vi "Distance calculation.vi"(8 "look up table":string[][](array[string])=[["", "1 0", "0 1", "1 -1", "-1 1", "1 -4", "-4 1", "2 0", "0 2", "2 -1", "-1 2", "2 -2", "-2 2", "3 0", "0 3", "3 -2", "-2 3", "3 -3", "-3 3", "4 0", "0 4", "4 -3", "-3 4", "4 -4", "-4 4", "-1 0", "0 -1", "-2 0", "0 -2", "-3 0", "0 -3", "-4 0", "0 -4", "-1 -2", "-2 -1", "-2 -3", "-3 -2", "-3 -4", "-4 -3", "-4 -1", "-1 -4"], ["-4", "2", "2", "2", "2", "1", "0", "4", "4", "4", "4", "4", "4", "4", "4", "4", "4", "4", "4", "2", "2", "2", "2", "1", "0", "3", "2", "5", "5", "3", "2", "0", "1", "4", "4", "4", "4", "1", "0", "0", "1"], ["-3", "4", "4", "4", "4", "4", "4", "4", "4", "4", "4", "4", "4", "2", "2", "2", "2", "1", "0", "2", "2", "1", "0", "2", "2", "5", "5", "3", "2", "0", "1", "3", "2", "4", "4", "1", "0", "0", "1", "4", "4"], ["-2", "4", "4", "4", "4", "4", "4", "2", "2", "2", "2", "1", "0", "2", "2", "1", "0", "2", "2", "4", "4", "4", "4", "4", "4", "3", "2", "0", "1", "3", "2", "5", "5", "1", "0", "0", "1", "4", "4", "4", "4"], ["-1", "2", "2", "1", "0", "2", "2", "2", "2", "1", "0", "2", "2", "4", "4", "4", "4", "4", "4", "4", "4", "4", "4", "4", "4", "0", "1", "3", "2", "5", "5", "3", "2", "0", "1", "4", "4", "4", "4", "1", "0"], ["0", "1", "0", "2", "2", "2", "2", "1", "0", "2", "2", "2", "2", "1", "0", "2", "2", "2", "2", "1", "0", "2", "2", "2", "2", "1", "0", "1", "0", "1", "0", "1", "0", "2", "2", "2", "2", "2", "2", "2", "2"], ["1", "0", "1", "0", "1", "0", "1", "3", "3", "3", "3", "3", "3", "5", "5", "5", "5", "5", "5", "3", "3", "3", "3", "3", "3", "2", "3", "4", "4", "4", "4", "2", "3", "3", "3", "5", "5", "3", "3", "2", "2"], ["2", "3", "3", "3", "3", "3", "3", "0", "1", "0", "1", "0", "1", "3", "3", "3", "3", "3", "3", "5", "5", "5", "5", "5", "5", "2", "3", "2", "3", "4", "4", "4", "4", "2", "2", "3", "3", "5", "5", "3", "3"], ["3", "5", "5", "5", "5", "5", "5", "3", "3", "3", "3", "3", "3", "0", "1", "0", "1", "0", "1", "3", "3", "3", "3", "3", "3", "4", "4", "2", "3", "2", "3", "4", "4", "3", "3", "2", "2", "3", "3", "5", "5"], ["4", "3", "3", "3", "3", "3", "3", "5", "5", "5", "5", "5", "5", "3", "3", "3", "3", "3", "3", "0", "1", "0", "1", "0", "1", "4", "4", "4", "4", "2", "3", "2", "3", "5", "5", "3", "3", "4", "4", "3", "3"]], 10 "cluster centers":string[](array[string])=["1 0 1", "2 0 2", "3 0 3", "4 0 4"], 11 "Patterns in":string[](array[string])=["0 4 0", "4 0 4", "0 4 0", "4 0 4", "0 4 0", "4 0 4", "0 4 0", "4 0 -2", "0 -2 3", "-2 3 0", "3 0 3", "0 3 0", "3 0 4", "0 4 0", "-2 0 1", "0 1 0", "1 0 -4", "0 -4 4", "-2 2 0", "2 0 -1", "0 -1 -4", "-1 -4 1", "-4 1 0", "1 0 3", "0 3 0", "-1 0 -1", "0 -1 2", "0 -1 1", "-1 1 0", "1 0 4", "0 4 0", "4 0 3", "0 3 -2", "3 -2 0", "-2 0 -2", "0 -2 3", "-2 3 -2", "3 -2 0", "-2 0 4", "0 4 0", "4 0 -2", "0 -2 2", "2 -1 0", "-1 0 4", "0 4 0", "4 0 2", "0 2 0", "2 0 -2", "0 -2 0", "1 -1 0", "-1 0 3", "0 3 0", "3 0 -4", "0 -4 4", "-4 4 -4", "4 -4 0", "2 -1 0", "-1 0 3", "0 3 -2", "3 -2 0", "-2 0 -3", "0 -3 0", "-3 0 3", "0 3 0", "3 0 -3", "0 -3 0", "0 4 0", "4 0 4", "0 4 -4", "4 -4 1", "-4 1 -1", "1 -1 0", "-1 0 -3", "0 -3 0", "-3 0 1", "0 1 -4", "1 -4 1", "-4 1 0", "1 0 4", "0 4 0", "4 0 -4", "0 -4 0", "-4 0 -4", "0 -4 4", "-4 4 -4", "4 -4 1", "0 -4 1", "-4 1 0", "1 0 -4", "0 -4 4", "0 4 0", "4 0 -2", "0 -2 2", "-2 2 -2", "2 -2 2", "-2 2 -2", "2 -2 2", "-2 2 -1", "2 -1 0", "-1 0 4", "0 4 0", "4 0 2", "0 2 0", "2 0 4", "0 4 0", "4 0 2", "0 2 -2", "2 -2 0", "-2 0 4", "1 0 -1", "0 -1 0", "-1 0 -1", "0 -1 0", "-1 0 1", "0 1 -1", "-2 2 -2", "2 -2 3", "1 0 -1", "0 -1 0", "-1 0 -1", "0 -1 2", "-1 2 0", "2 0 2", "0 2 -2", "2 -2 0", "-2 0 -4", "0 -4 0", "-2 2 0", "2 0 3", "0 3 -2", "3 -2 2", "1 -1 0", "-1 0 3", "0 4 0", "-2 0 1", "0 1 -4", "1 -4 0", "-4 0 -3", "0 -3 0", "1 0 -1", "0 -1 2", "-1 2 -1", "2 -1 1", "-1 1 -4", "-2 0 -1", "0 -1 1", "0 3 0", "3 0 3", "0 3 0", "3 0 3", "0 3 -2", "-4 0 -4", "0 -4 4", "0 4 0", "4 0 -4", "0 -4 0", "-4 0 -4", "-2 2 0", "2 0 4", "0 4 -4", "4 -4 0", "-4 0 2", "0 2 -2"]) -> (3 "Pattern (0) Distance data (1 to X) cluster (X+1) output":string[][](array[string]))   [LabVIEW 2013]
uses:
  cluster.ctl
panel:
  in  "15":string[](array[string])=["0 4 0 4 0 4 0 4 0 -2 3 0 3 0 4", "4 0 4 0 4 0 4 0 -2 3 0 3 0 4 0", "0 -1 1 0 4 0 3 -2 0 -2 3 -2 0 4 0", "-1 1 0 4 0 3 -2 0 -2 3 -2 0 4 0 -2", "1 0 4 0 3 -2 0 -2 3 -2 0 4 0 -2 2", "0 4 0 4 -4 1 -1 0 -3 0 1 -4 1 0 4", "4 0 4 -4 1 -1 0 -3 0 1 -4 1 0 4 0", "0 4 -4 1 -1 0 -3 0 1 -4 1 0 4 0 -4", "4 -4 1 -1 0 -3 0 1 -4 1 0 4 0 -4 0", "-4 1 -1 0 -3 0 1 -4 1 0 4 0 -4 0 -4", "1 -1 0 -3 0 1 -4 1 0 4 0 -4 0 -4 4", "-1 0 -3 0 1 -4 1 0 4 0 -4 0 -4 4 -4", "0 -3 0 1 -4 1 0 4 0 -4 0 -4 4 -4 1"]
  in  "14":string[](array[string])=["0 4 0 4 0 4 0 4 0 -2 3 0 3 0", "4 0 4 0 4 0 4 0 -2 3 0 3 0 4", "0 4 0 4 0 4 0 -2 3 0 3 0 4 0", "0 -1 1 0 4 0 3 -2 0 -2 3 -2 0 4", "-1 1 0 4 0 3 -2 0 -2 3 -2 0 4 0", "1 0 4 0 3 -2 0 -2 3 -2 0 4 0 -2", "0 4 0 3 -2 0 -2 3 -2 0 4 0 -2 2", "0 4 0 4 -4 1 -1 0 -3 0 1 -4 1 0", "4 0 4 -4 1 -1 0 -3 0 1 -4 1 0 4", "0 4 -4 1 -1 0 -3 0 1 -4 1 0 4 0", "4 -4 1 -1 0 -3 0 1 -4 1 0 4 0 -4", "-4 1 -1 0 -3 0 1 -4 1 0 4 0 -4 0", "1 -1 0 -3 0 1 -4 1 0 4 0 -4 0 -4", "-1 0 -3 0 1 -4 1 0 4 0 -4 0 -4 4", "0 -3 0 1 -4 1 0 4 0 -4 0 -4 4 -4", "-3 0 1 -4 1 0 4 0 -4 0 -4 4 -4 1", "-2 2 -1 0 4 0 2 0 4 0 2 -2 0 4"]
  in  "11":string[](array[string])=["0 4 0 4 0 4 0 4 0 -2 3", "4 0 4 0 4 0 4 0 -2 3 0", "0 4 0 4 0 4 0 -2 3 0 3", "4 0 4 0 4 0 -2 3 0 3 0", "0 4 0 4 0 -2 3 0 3 0 4", "4 0 4 0 -2 3 0 3 0 4 0", "0 -1 1 0 4 0 3 -2 0 -2 3", "-1 1 0 4 0 3 -2 0 -2 3 -2", "1 0 4 0 3 -2 0 -2 3 -2 0", "0 4 0 3 -2 0 -2 3 -2 0 4", "4 0 3 -2 0 -2 3 -2 0 4 0", "0 3 -2 0 -2 3 -2 0 4 0 -2", "3 -2 0 -2 3 -2 0 4 0 -2 2", "2 -1 0 3 -2 0 -3 0 3 0 -3", "-1 0 3 -2 0 -3 0 3 0 -3 0", "0 4 0 4 -4 1 -1 0 -3 0 1", "4 0 4 -4 1 -1 0 -3 0 1 -4", "0 4 -4 1 -1 0 -3 0 1 -4 1", "4 -4 1 -1 0 -3 0 1 -4 1 0", "-4 1 -1 0 -3 0 1 -4 1 0 4", "1 -1 0 -3 0 1 -4 1 0 4 0", "-1 0 -3 0 1 -4 1 0 4 0 -4", "0 -3 0 1 -4 1 0 4 0 -4 0", "-3 0 1 -4 1 0 4 0 -4 0 -4", "0 1 -4 1 0 4 0 -4 0 -4 4", "1 -4 1 0 4 0 -4 0 -4 4 -4", "-4 1 0 4 0 -4 0 -4 4 -4 1", "-2 2 -1 0 4 0 2 0 4 0 2", "2 -1 0 4 0 2 0 4 0 2 -2", "-1 0 4 0 2 0 4 0 2 -2 0", "0 4 0 2 0 4 0 2 -2 0 4", "1 0 -1 0 -1 2 0 2 -2 0 -4", "0 -1 0 -1 2 0 2 -2 0 -4 0"]
  in  "10":string[](array[string])=["0 4 0 4 0 4 0 4 0 -2", "4 0 4 0 4 0 4 0 -2 3", "0 4 0 4 0 4 0 -2 3 0", "4 0 4 0 4 0 -2 3 0 3", "0 4 0 4 0 -2 3 0 3 0", "4 0 4 0 -2 3 0 3 0 4", "0 4 0 -2 3 0 3 0 4 0", "0 -1 1 0 4 0 3 -2 0 -2", "-1 1 0 4 0 3 -2 0 -2 3", "1 0 4 0 3 -2 0 -2 3 -2", "0 4 0 3 -2 0 -2 3 -2 0", "4 0 3 -2 0 -2 3 -2 0 4", "0 3 -2 0 -2 3 -2 0 4 0", "3 -2 0 -2 3 -2 0 4 0 -2", "-2 0 -2 3 -2 0 4 0 -2 2", "2 -1 0 3 -2 0 -3 0 3 0", "-1 0 3 -2 0 -3 0 3 0 -3", "0 3 -2 0 -3 0 3 0 -3 0", "0 4 0 4 -4 1 -1 0 -3 0", "4 0 4 -4 1 -1 0 -3 0 1", "0 4 -4 1 -1 0 -3 0 1 -4", "4 -4 1 -1 0 -3 0 1 -4 1", "-4 1 -1 0 -3 0 1 -4 1 0", "1 -1 0 -3 0 1 -4 1 0 4", "-1 0 -3 0 1 -4 1 0 4 0", "0 -3 0 1 -4 1 0 4 0 -4", "-3 0 1 -4 1 0 4 0 -4 0", "0 1 -4 1 0 4 0 -4 0 -4", "1 -4 1 0 4 0 -4 0 -4 4", "-4 1 0 4 0 -4 0 -4 4 -4", "1 0 4 0 -4 0 -4 4 -4 1", "-2 2 -1 0 4 0 2 0 4 0", "2 -1 0 4 0 2 0 4 0 2", "-1 0 4 0 2 0 4 0 2 -2", "0 4 0 2 0 4 0 2 -2 0", "4 0 2 0 4 0 2 -2 0 4", "1 0 -1 0 -1 2 0 2 -2 0", "0 -1 0 -1 2 0 2 -2 0 -4", "-1 0 -1 2 0 2 -2 0 -4 0"]
  in  "9":string[](array[string])=["0 4 0 4 0 4 0 4 0", "4 0 4 0 4 0 4 0 -2", "0 4 0 4 0 4 0 -2 3", "4 0 4 0 4 0 -2 3 0", "0 4 0 4 0 -2 3 0 3", "4 0 4 0 -2 3 0 3 0", "0 4 0 -2 3 0 3 0 4", "4 0 -2 3 0 3 0 4 0", "-2 2 0 -1 -4 1 0 3 0", "0 -1 1 0 4 0 3 -2 0", "-1 1 0 4 0 3 -2 0 -2", "1 0 4 0 3 -2 0 -2 3", "0 4 0 3 -2 0 -2 3 -2", "4 0 3 -2 0 -2 3 -2 0", "0 3 -2 0 -2 3 -2 0 4", "3 -2 0 -2 3 -2 0 4 0", "-2 0 -2 3 -2 0 4 0 -2", "0 -2 3 -2 0 4 0 -2 2", "1 -1 0 3 0 -4 4 -4 0", "2 -1 0 3 -2 0 -3 0 3", "-1 0 3 -2 0 -3 0 3 0", "0 3 -2 0 -3 0 3 0 -3", "3 -2 0 -3 0 3 0 -3 0", "0 4 0 4 -4 1 -1 0 -3", "4 0 4 -4 1 -1 0 -3 0", "0 4 -4 1 -1 0 -3 0 1", "4 -4 1 -1 0 -3 0 1 -4", "-4 1 -1 0 -3 0 1 -4 1", "1 -1 0 -3 0 1 -4 1 0", "-1 0 -3 0 1 -4 1 0 4", "0 -3 0 1 -4 1 0 4 0", "-3 0 1 -4 1 0 4 0 -4", "0 1 -4 1 0 4 0 -4 0", "1 -4 1 0 4 0 -4 0 -4", "-4 1 0 4 0 -4 0 -4 4", "1 0 4 0 -4 0 -4 4 -4", "0 4 0 -4 0 -4 4 -4 1", "0 4 0 -2 2 -2 2 -2 2", "-2 2 -1 0 4 0 2 0 4", "2 -1 0 4 0 2 0 4 0", "-1 0 4 0 2 0 4 0 2", "0 4 0 2 0 4 0 2 -2", "4 0 2 0 4 0 2 -2 0", "0 2 0 4 0 2 -2 0 4", "1 0 -1 0 -1 2 0 2 -2", "0 -1 0 -1 2 0 2 -2 0", "-1 0 -1 2 0 2 -2 0 -4", "0 -1 2 0 2 -2 0 -4 0"]
  in  "8":string[](array[string])=["0 4 0 4 0 4 0 4", "4 0 4 0 4 0 4 0", "0 4 0 4 0 4 0 -2", "4 0 4 0 4 0 -2 3", "0 4 0 4 0 -2 3 0", "4 0 4 0 -2 3 0 3", "0 4 0 -2 3 0 3 0", "4 0 -2 3 0 3 0 4", "0 -2 3 0 3 0 4 0", "-2 2 0 -1 -4 1 0 3", "2 0 -1 -4 1 0 3 0", "0 -1 1 0 4 0 3 -2", "-1 1 0 4 0 3 -2 0", "1 0 4 0 3 -2 0 -2", "0 4 0 3 -2 0 -2 3", "4 0 3 -2 0 -2 3 -2", "0 3 -2 0 -2 3 -2 0", "3 -2 0 -2 3 -2 0 4", "-2 0 -2 3 -2 0 4 0", "0 -2 3 -2 0 4 0 -2", "-2 3 -2 0 4 0 -2 2", "1 -1 0 3 0 -4 4 -4", "-1 0 3 0 -4 4 -4 0", "2 -1 0 3 -2 0 -3 0", "-1 0 3 -2 0 -3 0 3", "0 3 -2 0 -3 0 3 0", "3 -2 0 -3 0 3 0 -3", "-2 0 -3 0 3 0 -3 0", "0 4 0 4 -4 1 -1 0", "4 0 4 -4 1 -1 0 -3", "0 4 -4 1 -1 0 -3 0", "4 -4 1 -1 0 -3 0 1", "-4 1 -1 0 -3 0 1 -4", "1 -1 0 -3 0 1 -4 1", "-1 0 -3 0 1 -4 1 0", "0 -3 0 1 -4 1 0 4", "-3 0 1 -4 1 0 4 0", "0 1 -4 1 0 4 0 -4", "1 -4 1 0 4 0 -4 0", "-4 1 0 4 0 -4 0 -4", "1 0 4 0 -4 0 -4 4", "0 4 0 -4 0 -4 4 -4", "4 0 -4 0 -4 4 -4 1", "0 4 0 -2 2 -2 2 -2", "4 0 -2 2 -2 2 -2 2", "-2 2 -1 0 4 0 2 0", "2 -1 0 4 0 2 0 4", "-1 0 4 0 2 0 4 0", "0 4 0 2 0 4 0 2", "4 0 2 0 4 0 2 -2", "0 2 0 4 0 2 -2 0", "2 0 4 0 2 -2 0 4", "1 0 -1 0 -1 0 1 -1", "1 0 -1 0 -1 2 0 2", "0 -1 0 -1 2 0 2 -2", "-1 0 -1 2 0 2 -2 0", "0 -1 2 0 2 -2 0 -4", "-1 2 0 2 -2 0 -4 0", "-2 2 0 4 -4 0 2 -2"]
  in  "7":string[](array[string])=["0 4 0 4 0 4 0", "4 0 4 0 4 0 4", "0 4 0 4 0 4 0", "4 0 4 0 4 0 -2", "0 4 0 4 0 -2 3", "4 0 4 0 -2 3 0", "0 4 0 -2 3 0 3", "4 0 -2 3 0 3 0", "0 -2 3 0 3 0 4", "-2 3 0 3 0 4 0", "-2 2 0 -1 -4 1 0", "2 0 -1 -4 1 0 3", "0 -1 -4 1 0 3 0", "0 -1 1 0 4 0 3", "-1 1 0 4 0 3 -2", "1 0 4 0 3 -2 0", "0 4 0 3 -2 0 -2", "4 0 3 -2 0 -2 3", "0 3 -2 0 -2 3 -2", "3 -2 0 -2 3 -2 0", "-2 0 -2 3 -2 0 4", "0 -2 3 -2 0 4 0", "-2 3 -2 0 4 0 -2", "3 -2 0 4 0 -2 2", "0 4 0 2 0 -2 0", "1 -1 0 3 0 -4 4", "-1 0 3 0 -4 4 -4", "0 3 0 -4 4 -4 0", "2 -1 0 3 -2 0 -3", "-1 0 3 -2 0 -3 0", "0 3 -2 0 -3 0 3", "3 -2 0 -3 0 3 0", "-2 0 -3 0 3 0 -3", "0 -3 0 3 0 -3 0", "0 4 0 4 -4 1 -1", "4 0 4 -4 1 -1 0", "0 4 -4 1 -1 0 -3", "4 -4 1 -1 0 -3 0", "-4 1 -1 0 -3 0 1", "1 -1 0 -3 0 1 -4", "-1 0 -3 0 1 -4 1", "0 -3 0 1 -4 1 0", "-3 0 1 -4 1 0 4", "0 1 -4 1 0 4 0", "1 -4 1 0 4 0 -4", "-4 1 0 4 0 -4 0", "1 0 4 0 -4 0 -4", "0 4 0 -4 0 -4 4", "4 0 -4 0 -4 4 -4", "0 -4 0 -4 4 -4 1", "0 4 0 -2 2 -2 2", "4 0 -2 2 -2 2 -2", "0 -2 2 -2 2 -2 2", "-2 2 -1 0 4 0 2", "2 -1 0 4 0 2 0", "-1 0 4 0 2 0 4", "0 4 0 2 0 4 0", "4 0 2 0 4 0 2", "0 2 0 4 0 2 -2", "2 0 4 0 2 -2 0", "0 4 0 2 -2 0 4", "1 0 -1 0 -1 0 1", "0 -1 0 -1 0 1 -1", "1 0 -1 0 -1 2 0", "0 -1 0 -1 2 0 2", "-1 0 -1 2 0 2 -2", "0 -1 2 0 2 -2 0", "-1 2 0 2 -2 0 -4", "2 0 2 -2 0 -4 0", "-2 0 1 -4 0 -3 0", "1 0 -1 2 -1 1 -4", "0 3 0 3 0 3 -2", "-2 2 0 4 -4 0 2", "2 0 4 -4 0 2 -2"]
  in  "6":string[](array[string])=["0 4 0 4 0 4", "4 0 4 0 4 0", "0 4 0 4 0 4", "4 0 4 0 4 0", "0 4 0 4 0 -2", "4 0 4 0 -2 3", "0 4 0 -2 3 0", "4 0 -2 3 0 3", "0 -2 3 0 3 0", "-2 3 0 3 0 4", "3 0 3 0 4 0", "-2 0 1 0 -4 4", "-2 2 0 -1 -4 1", "2 0 -1 -4 1 0", "0 -1 -4 1 0 3", "-1 -4 1 0 3 0", "0 -1 1 0 4 0", "-1 1 0 4 0 3", "1 0 4 0 3 -2", "0 4 0 3 -2 0", "4 0 3 -2 0 -2", "0 3 -2 0 -2 3", "3 -2 0 -2 3 -2", "-2 0 -2 3 -2 0", "0 -2 3 -2 0 4", "-2 3 -2 0 4 0", "3 -2 0 4 0 -2", "-2 0 4 0 -2 2", "0 4 0 2 0 -2", "4 0 2 0 -2 0", "1 -1 0 3 0 -4", "-1 0 3 0 -4 4", "0 3 0 -4 4 -4", "3 0 -4 4 -4 0", "2 -1 0 3 -2 0", "-1 0 3 -2 0 -3", "0 3 -2 0 -3 0", "3 -2 0 -3 0 3", "-2 0 -3 0 3 0", "0 -3 0 3 0 -3", "-3 0 3 0 -3 0", "0 4 0 4 -4 1", "4 0 4 -4 1 -1", "0 4 -4 1 -1 0", "4 -4 1 -1 0 -3", "-4 1 -1 0 -3 0", "1 -1 0 -3 0 1", "-1 0 -3 0 1 -4", "0 -3 0 1 -4 1", "-3 0 1 -4 1 0", "0 1 -4 1 0 4", "1 -4 1 0 4 0", "-4 1 0 4 0 -4", "1 0 4 0 -4 0", "0 4 0 -4 0 -4", "4 0 -4 0 -4 4", "0 -4 0 -4 4 -4", "-4 0 -4 4 -4 1", "0 -4 1 0 -4 4", "0 4 0 -2 2 -2", "4 0 -2 2 -2 2", "0 -2 2 -2 2 -2", "-2 2 -2 2 -2 2", "-2 2 -1 0 4 0", "2 -1 0 4 0 2", "-1 0 4 0 2 0", "0 4 0 2 0 4", "4 0 2 0 4 0", "0 2 0 4 0 2", "2 0 4 0 2 -2", "0 4 0 2 -2 0", "4 0 2 -2 0 4", "1 0 -1 0 -1 0", "0 -1 0 -1 0 1", "-1 0 -1 0 1 -1", "1 0 -1 0 -1 2", "0 -1 0 -1 2 0", "-1 0 -1 2 0 2", "0 -1 2 0 2 -2", "-1 2 0 2 -2 0", "2 0 2 -2 0 -4", "0 2 -2 0 -4 0", "-2 2 0 3 -2 2", "-2 0 1 -4 0 -3", "0 1 -4 0 -3 0", "1 0 -1 2 -1 1", "0 -1 2 -1 1 -4", "0 3 0 3 0 3", "3 0 3 0 3 -2", "0 4 0 -4 0 -4", "-2 2 0 4 -4 0", "2 0 4 -4 0 2", "0 4 -4 0 2 -2"]
  in  "4":string[](array[string])=["0 4 0 4", "4 0 4 0", "0 4 0 4", "4 0 4 0", "0 4 0 4", "4 0 4 0", "0 4 0 -2", "4 0 -2 3", "0 -2 3 0", "-2 3 0 3", "3 0 3 0", "0 3 0 4", "3 0 4 0", "-2 0 1 0", "0 1 0 -4", "1 0 -4 4", "-2 2 0 -1", "2 0 -1 -4", "0 -1 -4 1", "-1 -4 1 0", "-4 1 0 3", "1 0 3 0", "-1 0 -1 2", "0 -1 1 0", "-1 1 0 4", "1 0 4 0", "0 4 0 3", "4 0 3 -2", "0 3 -2 0", "3 -2 0 -2", "-2 0 -2 3", "0 -2 3 -2", "-2 3 -2 0", "3 -2 0 4", "-2 0 4 0", "0 4 0 -2", "4 0 -2 2", "2 -1 0 4", "0 4 0 2", "4 0 2 0", "0 2 0 -2", "2 0 -2 0", "1 -1 0 3", "-1 0 3 0", "0 3 0 -4", "3 0 -4 4", "0 -4 4 -4", "-4 4 -4 0", "2 -1 0 3", "-1 0 3 -2", "0 3 -2 0", "3 -2 0 -3", "-2 0 -3 0", "0 -3 0 3", "-3 0 3 0", "0 3 0 -3", "3 0 -3 0", "0 4 0 4", "4 0 4 -4", "0 4 -4 1", "4 -4 1 -1", "-4 1 -1 0", "1 -1 0 -3", "-1 0 -3 0", "0 -3 0 1", "-3 0 1 -4", "0 1 -4 1", "1 -4 1 0", "-4 1 0 4", "1 0 4 0", "0 4 0 -4", "4 0 -4 0", "0 -4 0 -4", "-4 0 -4 4", "0 -4 4 -4", "-4 4 -4 1", "0 -4 1 0", "-4 1 0 -4", "1 0 -4 4", "0 4 0 -2", "4 0 -2 2", "0 -2 2 -2", "-2 2 -2 2", "2 -2 2 -2", "-2 2 -2 2", "-2 2 -1 0", "2 -1 0 4", "-1 0 4 0", "0 4 0 2", "4 0 2 0", "0 2 0 4", "2 0 4 0", "0 4 0 2", "4 0 2 -2", "0 2 -2 0", "2 -2 0 4", "1 0 -1 0", "0 -1 0 -1", "-1 0 -1 0", "0 -1 0 1", "-1 0 1 -1", "-2 2 -2 3", "1 0 -1 0", "0 -1 0 -1", "-1 0 -1 2", "0 -1 2 0", "-1 2 0 2", "2 0 2 -2", "0 2 -2 0", "2 -2 0 -4", "-2 0 -4 0", "-2 2 0 3", "2 0 3 -2", "0 3 -2 2", "1 -1 0 3", "-2 0 1 -4", "0 1 -4 0", "1 -4 0 -3", "-4 0 -3 0", "1 0 -1 2", "0 -1 2 -1", "-1 2 -1 1", "2 -1 1 -4", "-2 0 -1 1", "0 3 0 3", "3 0 3 0", "0 3 0 3", "3 0 3 -2", "-4 0 -4 4", "0 4 0 -4", "4 0 -4 0", "0 -4 0 -4", "-2 2 0 4", "2 0 4 -4", "0 4 -4 0", "4 -4 0 2", "-4 0 2 -2"]
  in  "5":string[](array[string])=["0 4 0 4 0", "4 0 4 0 4", "0 4 0 4 0", "4 0 4 0 4", "0 4 0 4 0", "4 0 4 0 -2", "0 4 0 -2 3", "4 0 -2 3 0", "0 -2 3 0 3", "-2 3 0 3 0", "3 0 3 0 4", "0 3 0 4 0", "-2 0 1 0 -4", "0 1 0 -4 4", "-2 2 0 -1 -4", "2 0 -1 -4 1", "0 -1 -4 1 0", "-1 -4 1 0 3", "-4 1 0 3 0", "0 -1 1 0 4", "-1 1 0 4 0", "1 0 4 0 3", "0 4 0 3 -2", "4 0 3 -2 0", "0 3 -2 0 -2", "3 -2 0 -2 3", "-2 0 -2 3 -2", "0 -2 3 -2 0", "-2 3 -2 0 4", "3 -2 0 4 0", "-2 0 4 0 -2", "0 4 0 -2 2", "0 4 0 2 0", "4 0 2 0 -2", "0 2 0 -2 0", "1 -1 0 3 0", "-1 0 3 0 -4", "0 3 0 -4 4", "3 0 -4 4 -4", "0 -4 4 -4 0", "2 -1 0 3 -2", "-1 0 3 -2 0", "0 3 -2 0 -3", "3 -2 0 -3 0", "-2 0 -3 0 3", "0 -3 0 3 0", "-3 0 3 0 -3", "0 3 0 -3 0", "0 4 0 4 -4", "4 0 4 -4 1", "0 4 -4 1 -1", "4 -4 1 -1 0", "-4 1 -1 0 -3", "1 -1 0 -3 0", "-1 0 -3 0 1", "0 -3 0 1 -4", "-3 0 1 -4 1", "0 1 -4 1 0", "1 -4 1 0 4", "-4 1 0 4 0", "1 0 4 0 -4", "0 4 0 -4 0", "4 0 -4 0 -4", "0 -4 0 -4 4", "-4 0 -4 4 -4", "0 -4 4 -4 1", "0 -4 1 0 -4", "-4 1 0 -4 4", "0 4 0 -2 2", "4 0 -2 2 -2", "0 -2 2 -2 2", "-2 2 -2 2 -2", "2 -2 2 -2 2", "-2 2 -1 0 4", "2 -1 0 4 0", "-1 0 4 0 2", "0 4 0 2 0", "4 0 2 0 4", "0 2 0 4 0", "2 0 4 0 2", "0 4 0 2 -2", "4 0 2 -2 0", "0 2 -2 0 4", "1 0 -1 0 -1", "0 -1 0 -1 0", "-1 0 -1 0 1", "0 -1 0 1 -1", "1 0 -1 0 -1", "0 -1 0 -1 2", "-1 0 -1 2 0", "0 -1 2 0 2", "-1 2 0 2 -2", "2 0 2 -2 0", "0 2 -2 0 -4", "2 -2 0 -4 0", "-2 2 0 3 -2", "2 0 3 -2 2", "-2 0 1 -4 0", "0 1 -4 0 -3", "1 -4 0 -3 0", "1 0 -1 2 -1", "0 -1 2 -1 1", "-1 2 -1 1 -4", "0 3 0 3 0", "3 0 3 0 3", "0 3 0 3 -2", "0 4 0 -4 0", "4 0 -4 0 -4", "-2 2 0 4 -4", "2 0 4 -4 0", "0 4 -4 0 2", "4 -4 0 2 -2"]
  in  "cluster":u32
  out "position counts":T1[](array[typedef])
  out "Pattern (0) Distance data (1-4) cluster (5) output 2":string[](array[string])
  out "Cluster center graph":cluster{"XY Graph":cluster{dbl[], dbl[]}}[](array[cluster])
  out "Cluster graph":cluster{"XY Graph":cluster{dbl[], dbl[]}[]}[](array[cluster])
  out "Best cluster centers":string[](array[string])
  out "Elements in clusters":i32[](array[numeric])
  out "Best Pattern (0) Distance data (1 to X) cluster (X+1) output":string[][](array[string])
  out "Numeric":i32
  in  "stop":bool
  out "cluster centers old":string[](array[string])
  out "New cluster centers":string[](array[string])
  in  "milliseconds to wait":u32(slide) scale=0.0..1000.0
  out "elements":i32[](array[numeric])
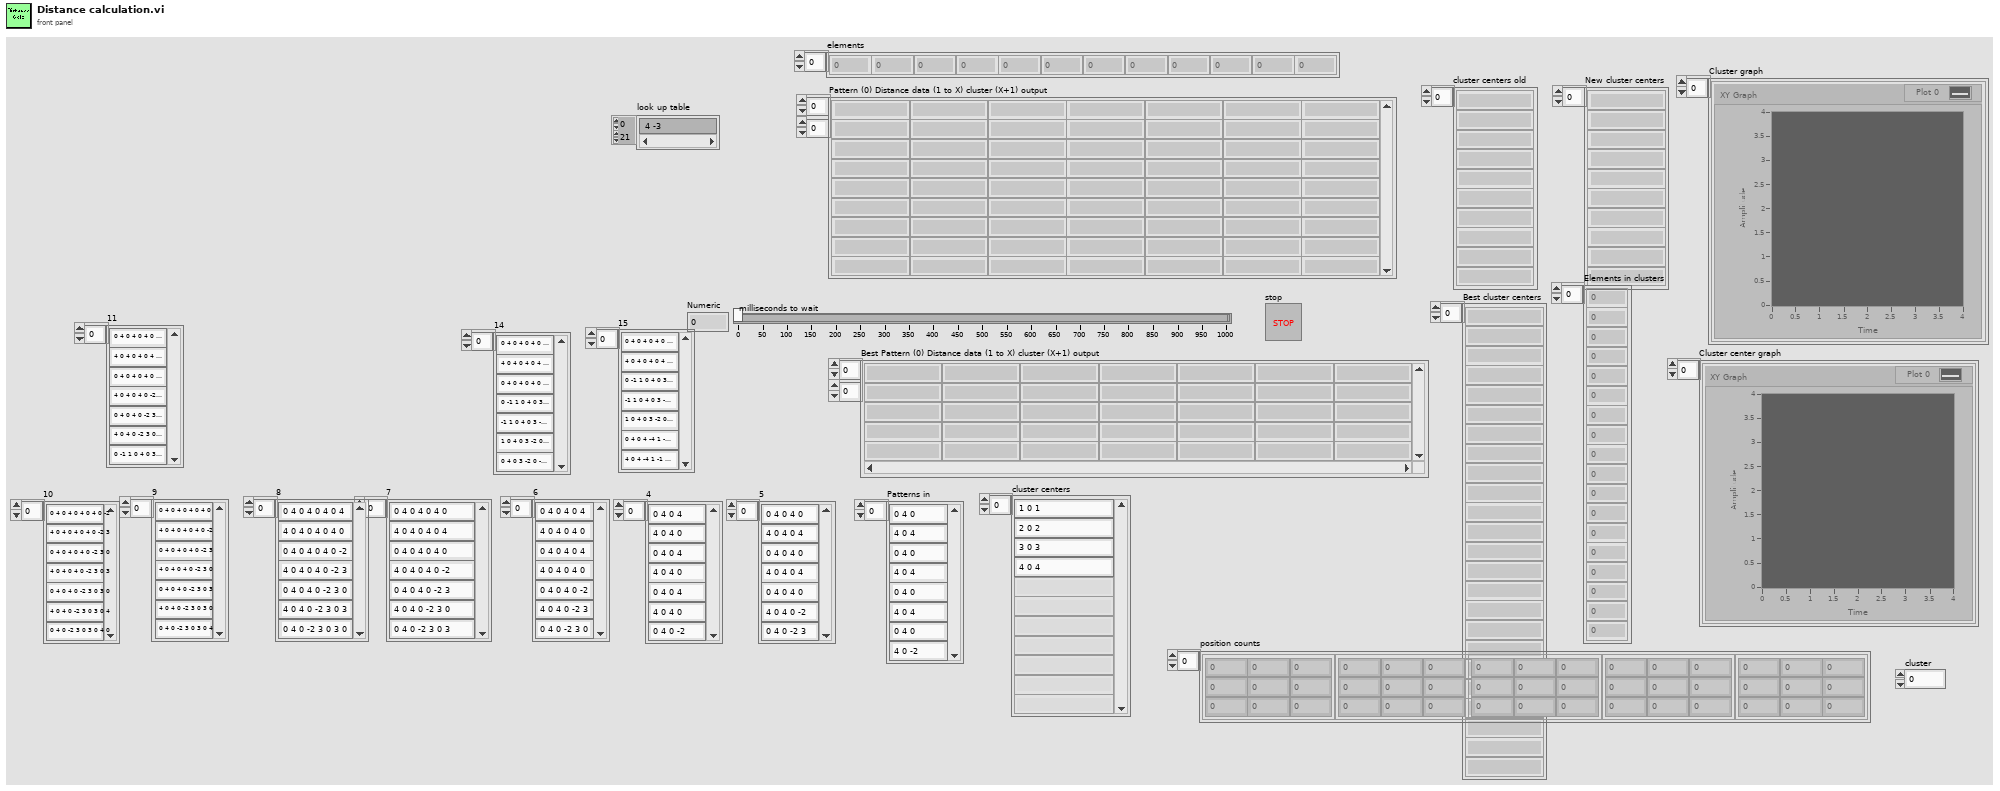
[diagram p1: front panel]
types:
  T1 = typedef "cluster.ctl" = cluster{dbl, dbl, dbl, dbl, dbl, dbl, dbl, dbl, dbl}
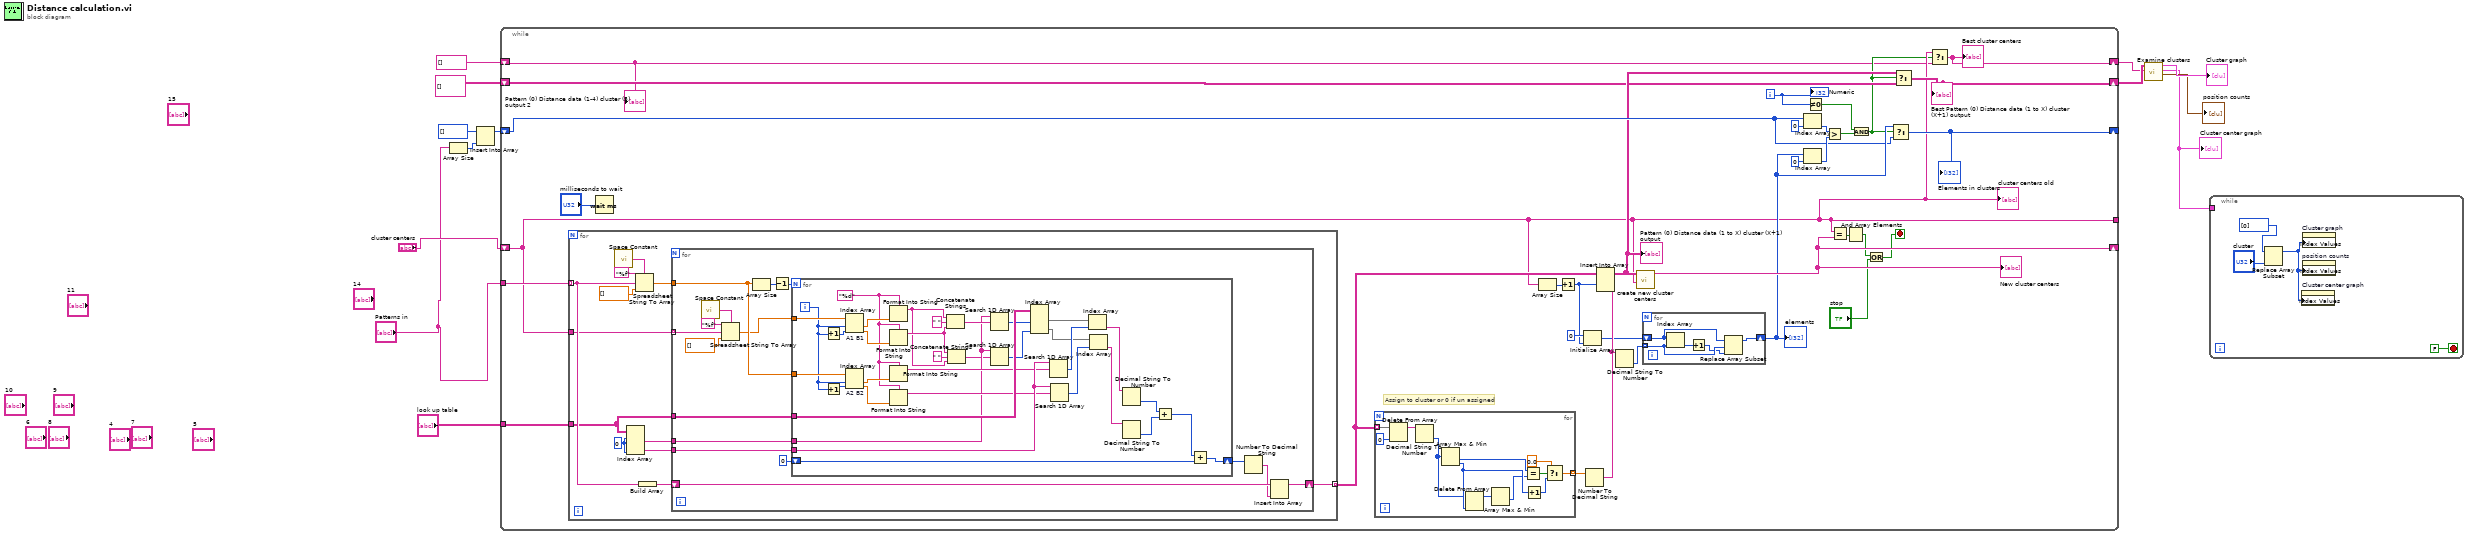
[diagram p0: block diagram]
diagram:
  n1 = Array Size(array="Patterns in") -> (size(s)=w10:i32)
  n2 = Insert Into Array(array=i32[] [] ("Array 2"), new element=w10) -> (w9:i32[])  [unwired: 1 in]
  n3 = while {
    tunnel: "look up table" -> [w46]
    shift-right: [w39] -> _
    shift-left: "cluster centers" -> [w19]
    tunnel: [w19] -> _
    tunnel: "Patterns in" -> [w38]
    shift-right: [w26] -> w7
    shift-left: string[][] [] ("Pattern (0) Distance data (1-4) cluster (5) output 2") -> [w24]
    shift-right: [w27] -> _
    shift-left: w9 -> [w28]
    shift-right: [w20] -> w6
    shift-left: string[] [] ("Pattern (0) Distance data (1-4) cluster (5) output 2") -> [w17]
    i -> [w23]
    stop <- w14 stop-if-true
    # "Assign to cluster or 0 if un assigned"
    n4 = for {
      tunnel: w38 -> [w67] mode=indexing
      tunnel: [w66] -> w44 mode=indexing
      tunnel: w19 -> [w65]
      tunnel: w46 -> [w64]
      w70 = 0 ("index")
      n5 = call <vilib>:"Space Constant.vi"() -> ("String"=w74:string)
      n6 = Index Array(array=w64, index (row) #1=w70, index (col) #2=w70) -> (element #1=w71:string[], element #2=w69:string[])  [unwired: 2 in]
      n7 = Spreadsheet String To Array(delimiter (Tab)=w74, format string="%f", spreadsheet string=w67, array type (2D Dbl)=dbl[] [] ("array 2")) -> (array=w72:dbl[])
      n8 = Build Array(w67) -> (w68:string[])
      n9 = for {
        tunnel: w72 -> [w89]
        tunnel: w65 -> [w85] mode=indexing
        tunnel: w71 -> [w83]
        tunnel: w69 -> [w82]
        tunnel: w64 -> [w81]
        shift-right: [w79] -> w66
        shift-left: w68 -> [w78]
        n10 = call <vilib>:"Space Constant.vi"() -> ("String"=w87:string)
        n11 = Spreadsheet String To Array(delimiter (Tab)=w87, format string="%f", spreadsheet string=w85, array type (2D Dbl)=dbl[] [] ("array 2")) -> (array=w84:dbl[])
        n12 = Array Size(array=w89) -> (size(s)=w91:i32)
        n13 = Decrement(x=w91) -> (x-1=w90:i32)
        n14 = for {
          N: w90 -> [_]
          tunnel: w89 -> [w125]
          tunnel: w84 -> [w122]
          tunnel: w83 -> [w102]
          tunnel: w82 -> [w111]
          tunnel: w81 -> [w116]
          shift-right: [w94] -> w77
          shift-left: 0 -> [w92]
          i -> [w121]
          w112 = "%d" ("format string")
          n15 = Increment(x=w121) -> (x+1=w123:i32)
          n16 = Increment(x=w121) -> (x+1=w124:i32)
          n17 = Index Array "A1 B1"(array=w122, index #1=w121, index #2=w123) -> (element #1=w119:dbl, element #2=w118:dbl)
          n18 = Index Array "A2 B2"(array=w125, index #1=w121, index #2=w124) -> (element #1=w114:dbl, element #2=w113:dbl)
          n19 = Format Into String(format string=w112, w119) -> (resulting string=w104:string)  [unwired: 2 in, 1 out]
          n20 = Format Into String(format string=w112, w118) -> (resulting string=w105:string)  [unwired: 2 in, 1 out]
          n21 = Format Into String(format string=w112, w114) -> (resulting string=w110:string)  [unwired: 2 in, 1 out]
          n22 = Format Into String(format string=w112, w113) -> (resulting string=w109:string)  [unwired: 2 in, 1 out]
          n23 = Concatenate Strings(w104, " " ("string"), w105) -> (w117:string)
          n24 = Concatenate Strings(w105, " " ("string"), w104) -> (w101:string)
          n25 = Search 1D Array(1D array=w102, element=w117) -> (index of element=w115:i32)  [unwired: 1 in]
          n26 = Search 1D Array(1D array=w102, element=w101) -> (index of element=w103:i32)  [unwired: 1 in]
          n27 = Index Array(array=w116, index (col) #1=w115, index (col) #2=w103) -> (element #1=w108:string[], element #2=w100:string[])  [unwired: 2 in]
          n28 = Search 1D Array(1D array=w111, element=w110) -> (index of element=w107:i32)  [unwired: 1 in]
          n29 = Search 1D Array(1D array=w111, element=w109) -> (index of element=w99:i32)  [unwired: 1 in]
          n30 = Index Array(array=w108, index=w107) -> (element=w98:string)
          n31 = Index Array(array=w100, index=w99) -> (element=w97:string)
          n32 = Decimal String To Number(string=w98) -> (number=w96:i32)  [unwired: 2 in, 1 out]
          n33 = Decimal String To Number(string=w97) -> (number=w95:i32)  [unwired: 2 in, 1 out]
          n34 = Add(x=w96, y=w95) -> (x+y=w93:i32)
          n35 = Add(x=w93, y=w92) -> (x+y=w94:i32)
        }
        n36 = Number To Decimal String(number=w77) -> (decimal integer string=w76:string)  [unwired: 1 in]
        n37 = Insert Into Array(array=w78, new element=w76) -> (w79:string[])  [unwired: 1 in]
      }
    }
    n38 = Wait (ms)(milliseconds to wait="milliseconds to wait") -> ()  [unwired: 1 out]
    n39 = for {
      tunnel: w44 -> [w63] mode=indexing
      tunnel: [w52] -> w45 mode=indexing
      n40 = Delete From Array(array=w63, index=0) -> (array with subset deleted=w61:string[])  [unwired: 1 in, 1 out]
      n41 = Decimal String To Number(string=w61) -> (number=w53:i32[])  [unwired: 2 in, 1 out]
      n42 = Array Max & Min(array=w53) -> (min value=w54:i32, min index (indices)=w57:i32)  [unwired: 2 out]
      n43 = Delete From Array(array=w53, index=w57) -> (array with subset deleted=w60:i32[])  [unwired: 1 in, 1 out]
      n44 = Array Max & Min(array=w60) -> (min value=w55:i32)  [unwired: 3 out]
      n45 = Equal?(x=w54, y=w55) -> (x = y?=w59:bool)
      n46 = Increment(x=w57) -> (x+1=w56:i32)
      n47 = Select(t=0.0, s=w59, f=w56) -> (s? t:f=w52:dbl)
    }
    n48 = Array Size(array=w19) -> (size(s)=w37:i32)
    n49 = Increment(x=w37) -> (x+1=w35:i32)
    n50 = Initialize Array(0 ("index"), w35) -> (w34:i32[])
    n51 = Number To Decimal String(number=w45) -> (decimal integer string=w43:string[])  [unwired: 1 in]
    n52 = Insert Into Array(array=w44, index (col)=w35, new element=w43) -> (w25:string[][])  [unwired: 1 in]
    "Pattern (0) Distance data (1 to X) cluster (X+1) output" <- w25
    n53 = Decimal String To Number(string=w43) -> (number=w42:i32[])  [unwired: 2 in, 1 out]
    n54 = call "create new cluster centers.vi"("Pattern (0) Distance data (1-4) cluster (5) output"=w25, "Old cluster centers"=w19) -> ("New cluster centers"=w39:string[])  [unwired: 8 in]
    "New cluster centers" <- w39
    n55 = for {
      tunnel: w42 -> [w49] mode=indexing
      shift-right: [w47] -> w29
      shift-left: w34 -> [w50]
      n56 = Index Array(array=w50, index=w49) -> (element=w51:i32)
      n57 = Increment(x=w51) -> (x+1=w48:i32)
      n58 = Replace Array Subset(array=w50, new element=w48, index=w49) -> (w47:i32[])
    }
    "elements" <- w29
    n59 = Index Array(array=w28, index=0) -> (element=w31:i32)
    n60 = Index Array(array=w29, index=0) -> (element=w30:i32)
    n61 = Not Equal To 0?(x=w23) -> (x != 0?=w21:bool)
    n62 = Greater?(x=w31, y=w30) -> (0:w22:bool)
    n63 = Equal?(x=w19, y=w39) -> (x = y?=w41:bool[])
    n64 = And Array Elements(Boolean array=w41) -> (logical AND=w15:bool)
    n65 = And(x=w21, y=w22) -> (x .and. y?=w18:bool)
    n66 = Or(x=w15, y="stop") -> (x .or. y?=w14:bool)
    n67 = Select(t=w29, s=w18, f=w28) -> (s? t:f=w27:i32[])
    "Elements in clusters" <- w27
    n68 = Select(t=w25, s=w18, f=w24) -> (s? t:f=w26:string[][])
    "Best Pattern (0) Distance data (1 to X) cluster (X+1) output" <- w26
    n69 = Select(t=w19, s=w18, f=w17) -> (s? t:f=w20:string[])
    "Best cluster centers" <- w20
    "cluster centers old" <- w19
    "Numeric" <- w23
    "Pattern (0) Distance data (1-4) cluster (5) output 2" <- w17
  }
  n70 = call "Examine clusters.vi"("Cluster centers"=w6, "Pattern (0) Distance data (1 to X) cluster (X+1) output"=w7) -> ("position counts"=→"position counts":T1[], "Cluster center graph"=w3:cluster{"XY Graph":cluster{dbl[], dbl[]}}[], "Cluster graph"=→"Cluster graph":cluster{"XY Graph":cluster{dbl[], dbl[]}[]}[])  [unwired: 7 in]
  "Cluster center graph" <- w3
  n71 = while {
    tunnel: w3 -> [_]
    stop <- FALSE stop-if-true
    n72 = Replace Array Subset(array=u32[] [0] ("Index Values"), new element="cluster") -> (w126:u32[])  [unwired: 1 in]
    n73 = property on="Cluster center graph" class="Arr (strict)"("Index Values"=w126) -> ()  [unwired: 2 in, 2 out]
    n74 = property on="Cluster graph" class="Arr (strict)"("Index Values"=w126) -> ()  [unwired: 2 in, 2 out]
    n75 = property on="position counts" class="Arr (strict)"("Index Values"=w126) -> ()  [unwired: 2 in, 2 out]
  }
